vi "Report.vi"() -> ()   [LabVIEW 2018]
uses:
  <vilib>/Utility/file.llb/Read Delimited Spreadsheet (string).vi
panel:
  in  "result":string
  in  "Search":bool
  in  "关键字":string
  in  "Listbox":i32(listbox)
  in  "Multicolumn Listbox":i32(listbox)
  # "测试报表查询"
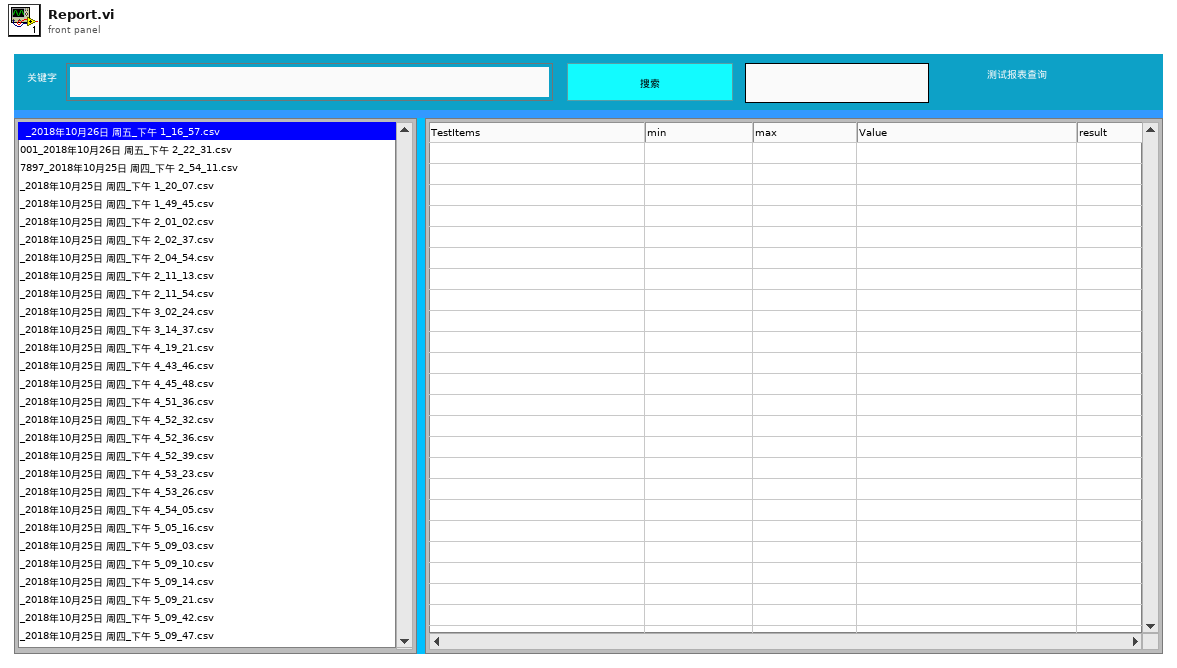
[diagram p1: front panel]
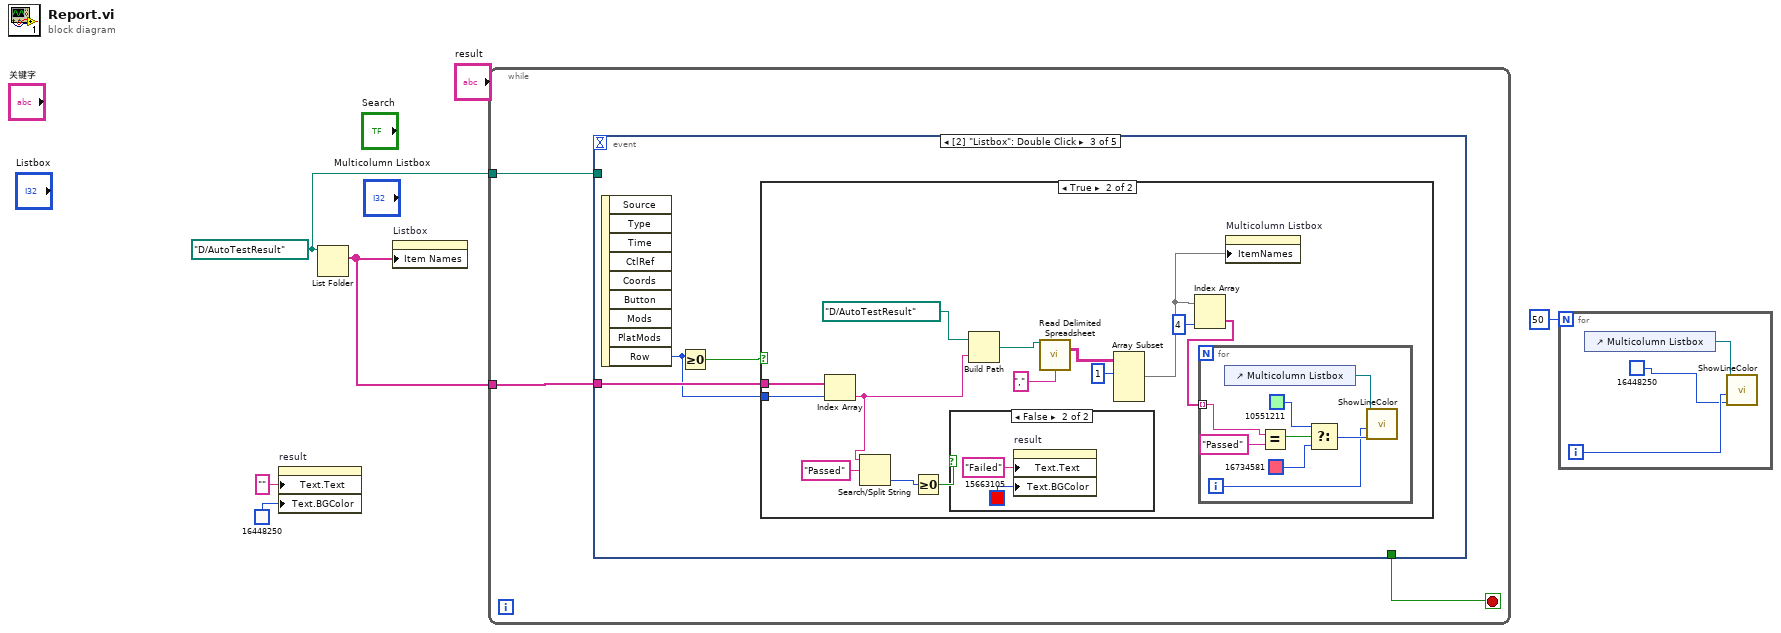
[diagram p0: block diagram]
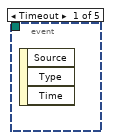
[diagram p2: hidden frame]
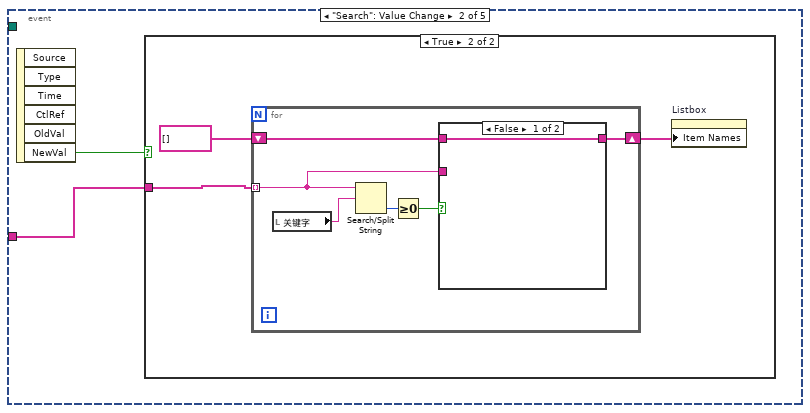
[diagram p3: hidden frame]
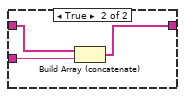
[diagram p5: hidden frame]
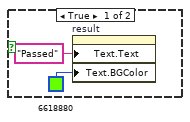
[diagram p7: hidden frame]
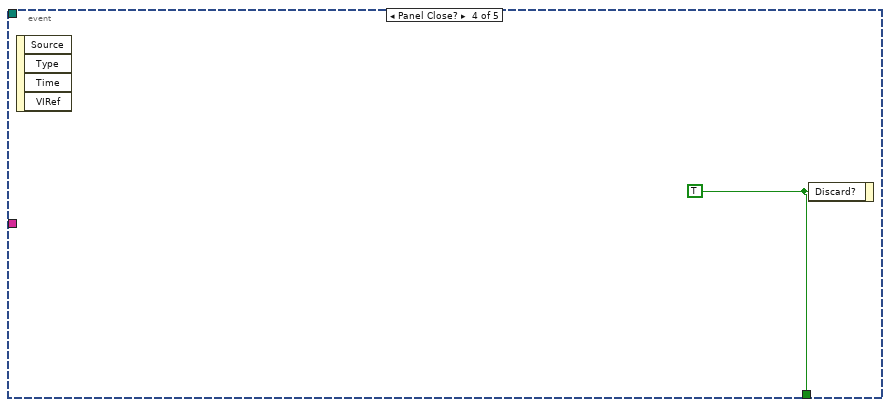
[diagram p8: hidden frame]
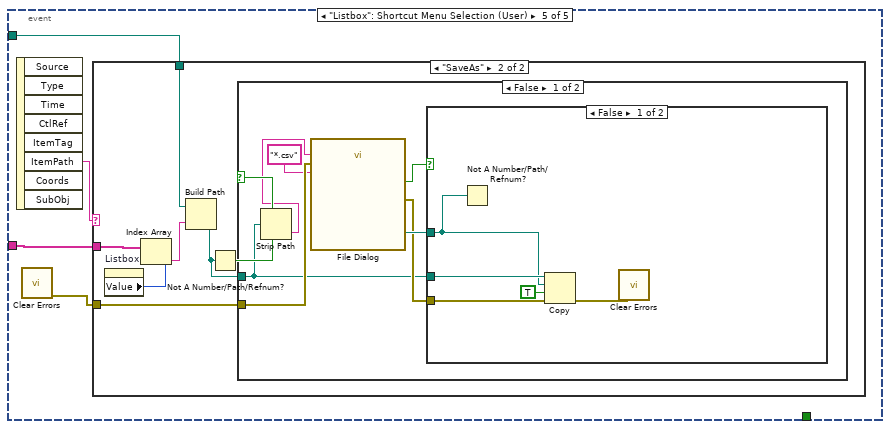
[diagram p9: hidden frame]
diagram:
  w4 = path "D:/AutoTestResult" ("path")
  n1 = property on="result" class="Str"("Text.Text"="", "Text.BGColor"=u32 16448250) -> ()  [unwired: 2 in, 2 out]
  n2 = List Folder(path=w4) -> (filenames=w5:string[])  [unwired: 3 in, 3 out]
  n3 = property on="Listbox" class="LstBox (strict)"("Item Names"=w5) -> ()  [unwired: 2 in, 2 out]
  n4 = while {
    tunnel: w5 -> [w8]
    tunnel: w4 -> [w6]
    stop <- w7 stop-if-true
    n5 = event shown="[2] \"Listbox\": Double Click" {
      selector: _ -> [_ _ _ _ _]
      dyn-events: _ -> [_ _ _ _ _]
      timeout: _ -> [_ _ _ _ _]
      tunnel: w8 -> [_ w9 w25 _ w56]
      tunnel: [_ _ _ w53 _] -> w7
      tunnel: w6 -> [_ _ _ _ w54]
      event Timeout {
        n6 = event-data() -> ()  [unwired: 1 in, 3 out]
      }
      event "Search": Value Change {
        n7 = event-data() -> ("NewVal"=w10:bool)  [unwired: 1 in, 5 out]
        n8 = case shown="True" w10 {
          tunnel: w9 -> [_ w13]
          frame False {
          }
          frame True {
            n9 = for {
              tunnel: w13 -> [w15] mode=indexing
              shift-right: [w14] -> w11
              shift-left: string[] [] -> [w16]
              n10 = local read "关键字"() -> (w19:string)
              n11 = Search/Split String(string=w15, search string/char (-)=w19) -> (offset of match=w18:i32)  [unwired: 1 in, 2 out]
              n12 = Greater Or Equal To 0?(x=w18) -> (x >= 0?=w17:bool)
              n13 = case shown="False" w17 {
                tunnel: w16 -> [w20 w23]
                tunnel: w15 -> [_ w22]
                tunnel: [w20 w21] -> w14
                frame False {
                }
                frame True {
                  n14 = Build Array (concatenate)(w23, w22) -> (w21:string[])
                }
              }
            }
            n15 = property on="Listbox" class="LstBox (strict)"("Item Names"=w11) -> ()  [unwired: 2 in, 2 out]
          }
        }
      }
      event "Listbox": Double Click {
        n16 = event-data() -> ("Row"=w24:i32)  [unwired: 1 in, 8 out]
        n17 = Greater Or Equal To 0?(x=w24) -> (x >= 0?=w26:bool)
        n18 = case shown="True" w26 {
          tunnel: w25 -> [_ w39]
          tunnel: w24 -> [_ w38]
          frame False {
          }
          frame True {
            n19 = Index Array(array=w39, index=w38) -> (element=w33:string)
            n20 = Search/Split String(string=w33, search string/char (-)="Passed") -> (offset of match=w31:i32)  [unwired: 1 in, 2 out]
            n21 = Greater Or Equal To 0?(x=w31) -> (x >= 0?=w30:bool)
            n22 = case shown="False" w30 {
              frame True {
                n23 = property on="result" class="Str"("Text.Text"="Passed", "Text.BGColor"=u32 6618880) -> ()  [unwired: 2 in, 2 out]
              }
              frame False {
                n24 = property on="result" class="Str"("Text.Text"="Failed", "Text.BGColor"=u32 15663105) -> ()  [unwired: 2 in, 2 out]
              }
            }
            n25 = Build Path(base path=path "D:/AutoTestResult" ("path"), name or relative path=w33) -> (appended path=w37:path)
            n26 = call-poly <vilib>:"Read Delimited Spreadsheet.vi"("file path (dialog if empty)"=w37, "delimiter (\\t)"="," ("delimiter (\\t)")) -> ("all rows"=w35:string[][])  [unwired: 8 in, 5 out]
            n27 = Array Subset(array=w35, index (row)=1 ("index")) -> (w29:string[][])  [unwired: 3 in]
            n28 = Index Array(array=w29, index (col)=4 ("disabled index (col)")) -> (element=w27:string[])  [unwired: 1 in]
            n29 = for {
              tunnel: w27 -> [w43] mode=indexing
              i -> [w42]
              n30 = control-ref of="Multicolumn Listbox"() -> (w41:refnum<vi>)
              n31 = Equal?(x=w43, y="Passed") -> (x = y?=w46:bool)
              n32 = Select(t=u32 10551211, s=w46, f=u32 16734581) -> (s? t:f=w44:u32)
              n33 = call "ShowLineColor.vi"("ColorIn"=w44, "TestingIndex"=w42, "MulticolumnListbox in"=w41) -> ()  [unwired: 9 in]
            }
            n34 = property on="Multicolumn Listbox" class="MCListbox (strict)"("ItemNames"=w29) -> ()  [unwired: 2 in, 2 out]
          }
        }
      }
      event Panel Close? {
        w53 = TRUE ("Discard?")
        n35 = event-data() -> ()  [unwired: 1 in, 4 out]
        n36 = event-data("Discard?"=w53) -> ()  [unwired: 1 in, 1 out]
      }
      event "Listbox": Shortcut Menu Selection (User) {
        n37 = event-data() -> ("ItemPath"=w57:string)  [unwired: 1 in, 7 out]
        n38 = call <vilib>:"Clear Errors.vi"() -> ("error out"=w55:errorcluster)  [unwired: 6 in, 1 out]
        n39 = case shown="\"SaveAs\"" w57 {
          tunnel: w56 -> [_ w64]
          tunnel: w55 -> [_ w61]
          tunnel: w54 -> [_ w60]
          frame "False", Default {
          }
          frame "SaveAs" {
            n40 = property on="Listbox" class="LstBox (strict)"() -> ("Value"=w63:i32)  [unwired: 2 in, 2 out]
            n41 = Index Array(array=w64, index=w63) -> (element=w59:string)
            n42 = Build Path(base path=w60, name or relative path=w59) -> (appended path=w58:path)
            n43 = Not A Number/Path/Refnum?(number/path/refnum=w58) -> (NaN/Path/Refnum?=w62:bool)
            n44 = case shown="False" w62 {
              tunnel: w58 -> [w67 _]
              tunnel: w61 -> [w70 _]
              frame False {
                n45 = Strip Path(path=w67) -> (name=w66:string)  [unwired: 1 out]
                n46 = call "File Dialog"("default name"=w66, "error in"=w70, "pattern (all files)"="*.csv" ("default name")) -> ("selected path"=w71:path, "cancelled"=w65:bool, "error out"=w69:errorcluster)  [unwired: 9 in, 1 out]
                n47 = case shown="False" w65 {
                  tunnel: w67 -> [w76 _]
                  tunnel: w71 -> [w74 _]
                  tunnel: w69 -> [w75 _]
                  frame False {
                    n48 = Not A Number/Path/Refnum?(number/path/refnum=w74) -> ()  [unwired: 1 out]
                    n49 = Copy(8:w75, 9:TRUE ("overwrite (F)"), 10:w74, 11:w76) -> (0:w73:errorcluster)  [unwired: 1 in, 2 out]
                    n50 = call <vilib>:"Clear Errors.vi"("error in (no error)"=w73) -> ()  [unwired: 5 in, 2 out]
                  }
                  frame True {
                  }
                }
              }
              frame True {
              }
            }
          }
        }
      }
    }
  }
  n51 = for {
    N: 50 -> [_]
    i -> [w79]
    n52 = control-ref of="Multicolumn Listbox"() -> (w78:refnum<vi>)
    n53 = call "ShowLineColor.vi"("ColorIn"=u32 16448250, "TestingIndex"=w79, "MulticolumnListbox in"=w78) -> ()  [unwired: 9 in]
  }
